vi "Stop Core.vi"(10 "final error code":i32, 11 "Driver-Logical in":refnum<class "Driver.lvclass">) -> (3 "Driver-Logical out":refnum<class "Driver.lvclass">)   [LabVIEW 2013, in "Logical Systems.lvlib" / "Driver.lvlib" / "Driver.lvclass"]
doc: "(<B>Filename</B>: Actor Framework.lvlib:Actor.lvclass:Stop Core.vi)\n\nDefines what the actor does before it stops. Use the <B>final error code</B> input to determine whether the actor shut down in response to an error.\n\nBy default, this method does nothing. A descendant class may override it to define behavior, such as shutting down any processes the actor initiated in its override of the Actor Core method."
uses:
  Driver.lvclass
  Robot Actors/System Actor/System Actor Class/System Actor.lvclass
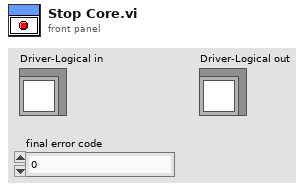
[diagram p1: front panel]
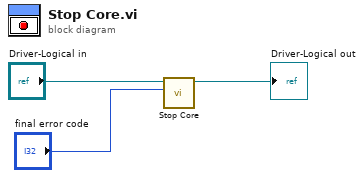
[diagram p0: block diagram]
diagram:
  n1 = call-parent "Stop Core.vi"("final error code"="final error code", "System Actor in"="Driver-Logical in") -> ("System Actor out"=→"Driver-Logical out":refnum<class "Driver.lvclass">)  [unwired: 9 in]
